vi "CONF HW card digital config.vi"(8 "error in (no error)":errorcluster, 9 "Config serial in":bool[][](array[boolean]), 10 "DATA task in":refnum<k21>, 11 "Enable task in":refnum<k21>) -> (0 "error out":errorcluster, 1 "Config serial out":bool[][](array[boolean]), 2 "DATA task out":refnum<k21>, 3 "Enable task out":refnum<k21>, 4 "config bits":i32)   [LabVIEW 2013]
doc: "Konfiguruje sprzetowa przejsciowke\nwysylajac sygnal do rejestrow przesownych"
uses:
  <vilib>/DAQmx/write.llb/DAQmx Write (Digital Bool 1Line 1Point).vi
  <vilib>/DAQmx/write.llb/DAQmx Write (Digital 1D Bool NChan 1Samp 1Line).vi
  <vilib>/DAQmx/miscellaneous.llb/DAQmx Fill In Error Info.vi
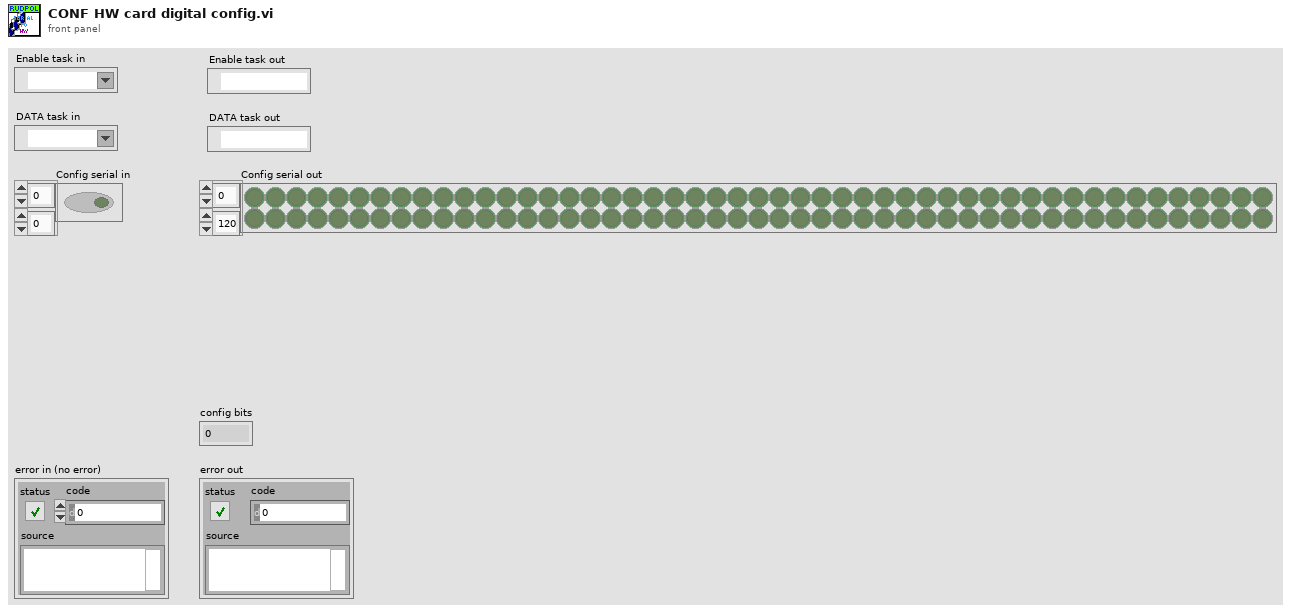
[diagram p1: front panel]
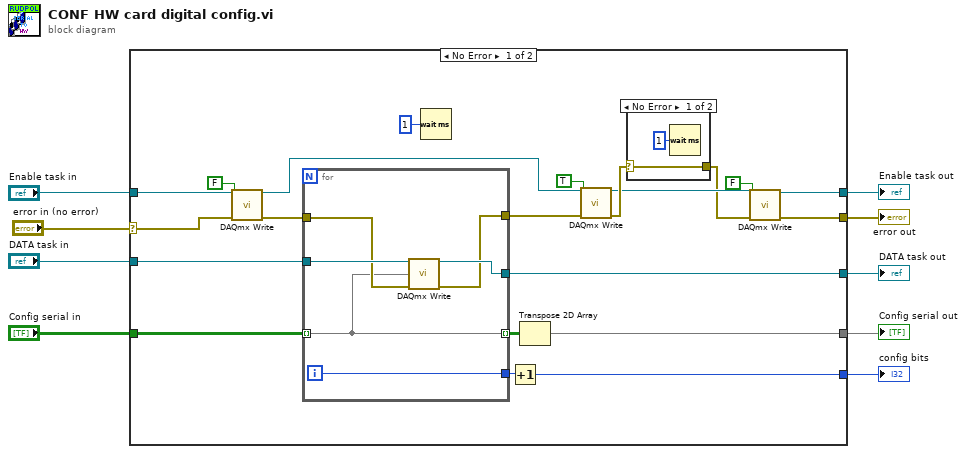
[diagram p0: block diagram]
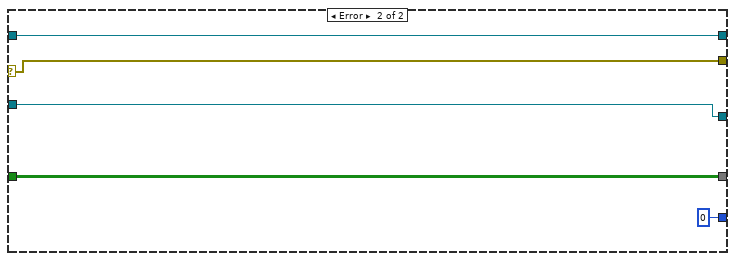
[diagram p3: hidden frame]
diagram:
  n1 = case shown="No Error" "error in (no error)" {
    selector: "error in (no error)" -> [w11 w43]
    tunnel: [w30 w43] -> w9
    tunnel: [w29 w41] -> w8
    tunnel: "Enable task in" -> [w26 w44]
    tunnel: "DATA task in" -> [w25 w42]
    tunnel: [w24 w42] -> w5
    tunnel: [w18 w44] -> w4
    tunnel: [w13 0] -> w3
    tunnel: "Config serial in" -> [w12 w41]
    frame No Error {
      n2 = call-poly <vilib>:"DAQmx Write.vi"("task/channels in"=w26, "data"=FALSE, "error in"=w11) -> ("task out"=w20:refnum<k21>, "error out"=w23:errorcluster)  [unwired: 10 in, 1 out]
      n3 = for {
        tunnel: w25 -> [w39]
        tunnel: [w38] -> w24
        tunnel: w23 -> [w37]
        tunnel: [w35] -> w21
        tunnel: [w36] -> w14
        tunnel: w12 -> [w34] mode=indexing
        tunnel: [w34] -> w28 mode=indexing
        i -> [w36]
        n4 = call-poly <vilib>:"DAQmx Write.vi"("task/channels in"=w39, "data"=w34, "error in"=w37) -> ("task out"=w38:refnum<k21>, "error out"=w35:errorcluster)  [unwired: 10 in, 1 out]
      }
      n5 = Wait (ms)(milliseconds to wait=u32 1) -> ()  [unwired: 1 out]
      n6 = Increment(x=w14) -> (x+1=w13:i32)
      n7 = Transpose 2D Array(2D array=w28) -> (transposed array=w29:bool[][])
      n8 = call-poly <vilib>:"DAQmx Write.vi"("task/channels in"=w20, "data"=TRUE, "error in"=w21) -> ("task out"=w19:refnum<k21>, "error out"=w27:errorcluster)  [unwired: 10 in, 1 out]
      n9 = case shown="No Error" w27 {
        selector: w27 -> [w32 w33]
        tunnel: [w32 w33] -> w15
        frame No Error {
          n10 = Wait (ms)(milliseconds to wait=u32 1) -> ()  [unwired: 1 out]
        }
        frame Error {
        }
      }
      n11 = call-poly <vilib>:"DAQmx Write.vi"("task/channels in"=w19, "data"=FALSE, "error in"=w15) -> ("task out"=w18:refnum<k21>, "error out"=w30:errorcluster)  [unwired: 10 in, 1 out]
    }
    frame Error {
    }
  }
  "config bits" <- w3
  "Config serial out" <- w8
  "error out" <- w9
  "DATA task out" <- w5
  "Enable task out" <- w4
